vi "I2C Communication.vi"(8 "error in":errorcluster) -> ()   [LabVIEW 2015]
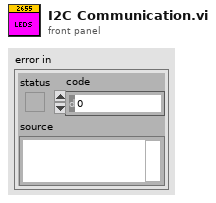
[diagram p1: front panel]
types:
  T1 = typedef "WPI_I2CDevRef.ctl" = cluster{"DevStatus":errorcluster, "Device Address":u8, "Handle":i32, "I2C Bus":T2}
  T2 = typedef "i2c_bus.ctl" = enum16{"I2C On-Board", "I2C MXP", "Invalid"}
  T3 = cluster{"I2CDevRef":T1, "error out":errorcluster}
  T4 = typedef "WPI_DriverStationAllianceInfo.ctl" = enum16{"Red", "Blue", "Invalid"}
  T5 = typedef "WPI_DriverStationRobotMode2.ctl" = enum16{"Autonomous Disabled", "Autonomous Enabled", "Teleop Disabled", "Teleop Enabled", "Disconnected", "Finish", "Test Disabled", "Test Enabled", "Emergency Stopped"}
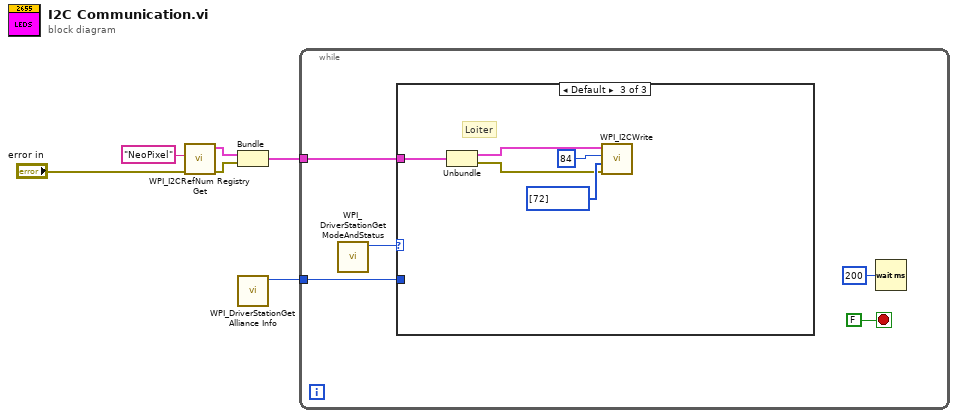
[diagram p0: block diagram]
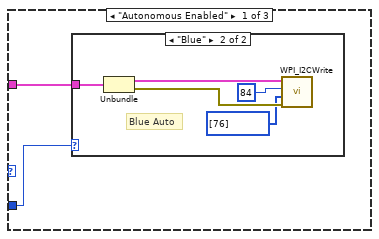
[diagram p2: hidden frame]
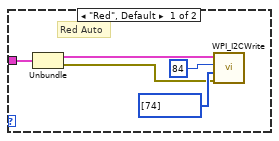
[diagram p3: hidden frame]
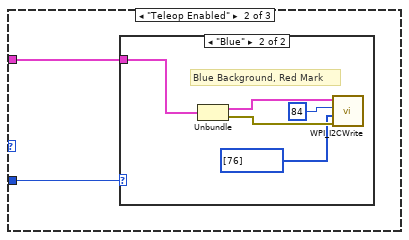
[diagram p4: hidden frame]
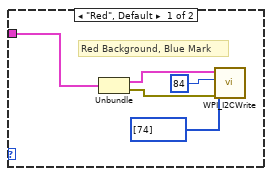
[diagram p5: hidden frame]
diagram:
  n1 = call <vilib>:"WPI_I2CRefNum Registry Get.vi"("error in (no error)"="error in", "refnum name"="NeoPixel") -> ("error out"=w6:errorcluster, "I2CDevRef"=w5:T1)  [unwired: 8 in]
  n2 = Bundle("I2CDevRef"=w5, "error out"=w6) -> (w3:T3)  [unwired: 1 in]
  n3 = call <vilib>:"WPI_DriverStationGet Alliance Info.vi"() -> ("Alliance"=w2:T4)  [unwired: 10 in, 1 out]
  n4 = while {
    tunnel: w3 -> [w9]
    tunnel: w2 -> [w7]
    stop <- FALSE stop-if-true
    n5 = call <vilib>:"WPI_DriverStationGetModeAndStatus.vi"() -> ("Robot Mode"=w8:T5)  [unwired: 10 in, 1 out]
    n6 = case shown="Default" w8 {
      tunnel: w9 -> [w13 w25 w36]
      tunnel: w7 -> [w12 w24 _]
      frame "Autonomous Enabled" {
        n7 = case shown="\"Blue\"" w12 {
          tunnel: w13 -> [w16 w19]
          frame "Red", Default {
            # "Red Auto"
            n8 = Unbundle(w16) -> ("I2CDevRef"=w15:T1, "error out"=w14:errorcluster)
            n9 = call <vilib>:"WPI_I2CWrite.vi"("error in (no error)"=w14, "I2CDataToSend"=u8[] [74], "I2CRegister"=u8 84, "I2CDevRef"=w15) -> ()  [unwired: 6 in, 2 out]
          }
          frame "Blue" {
            # "Blue Auto"
            n10 = Unbundle(w19) -> ("I2CDevRef"=w22:T1, "error out"=w23:errorcluster)
            n11 = call <vilib>:"WPI_I2CWrite.vi"("error in (no error)"=w23, "I2CDataToSend"=u8[] [76], "I2CRegister"=u8 84, "I2CDevRef"=w22) -> ()  [unwired: 6 in, 2 out]
          }
        }
      }
      frame "Teleop Enabled" {
        n12 = case shown="\"Blue\"" w24 {
          tunnel: w25 -> [w29 w32]
          frame "Red", Default {
            # "Red Background, Blue Mark"
            n13 = Unbundle(w29) -> ("I2CDevRef"=w28:T1, "error out"=w27:errorcluster)
            n14 = call <vilib>:"WPI_I2CWrite.vi"("error in (no error)"=w27, "I2CDataToSend"=u8[] [74], "I2CRegister"=u8 84, "I2CDevRef"=w28) -> ()  [unwired: 6 in, 2 out]
          }
          frame "Blue" {
            # "Blue Background, Red Mark"
            n15 = Unbundle(w32) -> ("I2CDevRef"=w34:T1, "error out"=w33:errorcluster)
            n16 = call <vilib>:"WPI_I2CWrite.vi"("error in (no error)"=w33, "I2CDataToSend"=u8[] [76], "I2CRegister"=u8 84, "I2CDevRef"=w34) -> ()  [unwired: 6 in, 2 out]
          }
        }
      }
      frame Default {
        # "Loiter"
        n17 = Unbundle(w36) -> ("I2CDevRef"=w38:T1, "error out"=w37:errorcluster)
        n18 = call <vilib>:"WPI_I2CWrite.vi"("error in (no error)"=w37, "I2CDataToSend"=u8[] [72], "I2CRegister"=u8 84, "I2CDevRef"=w38) -> ()  [unwired: 6 in, 2 out]
      }
    }
    n19 = Wait (ms)(milliseconds to wait=u32 200) -> ()  [unwired: 1 out]
  }
